vi "Calcy.vi"() -> ()   [LabVIEW 2025]
panel:
  in  "CLR":bool
  out "String":string
  in  "Keypad":T1
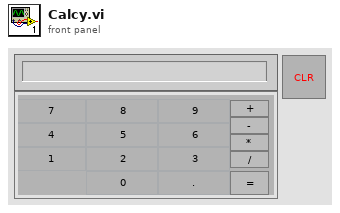
[diagram p1: front panel]
types:
  T1 = cluster{"0":bool, "1":bool, "2":bool, "3":bool, "4":bool, "5":bool, "6":bool, "7":bool, "8":bool, "9":bool, "decipoint":bool, "Add":bool, "Sub 3":bool, "Mul":bool, "Div":bool, "Equ":bool}
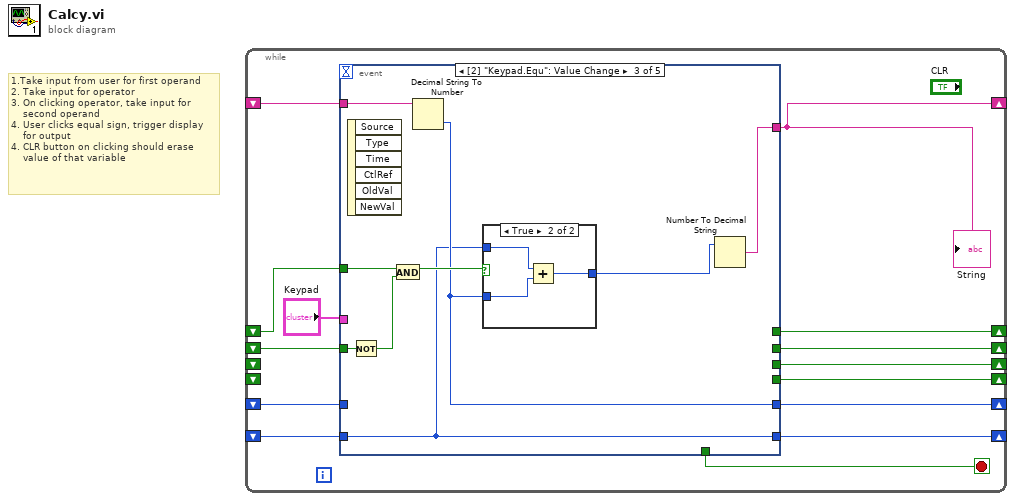
[diagram p0: block diagram]
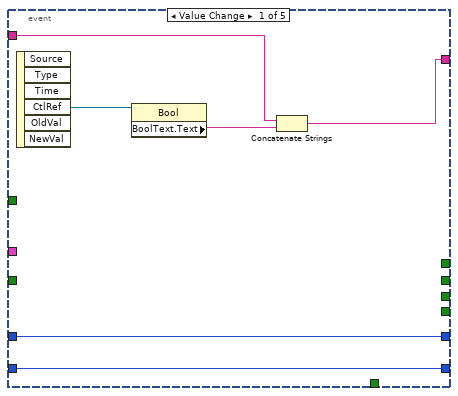
[diagram p2: hidden frame]
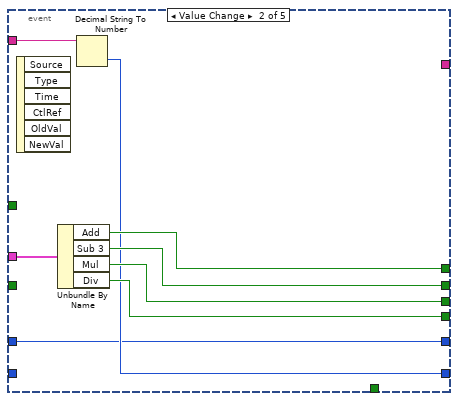
[diagram p3: hidden frame]
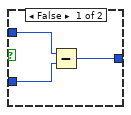
[diagram p4: hidden frame]
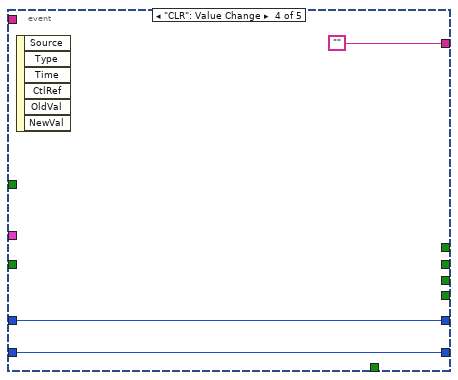
[diagram p5: hidden frame]
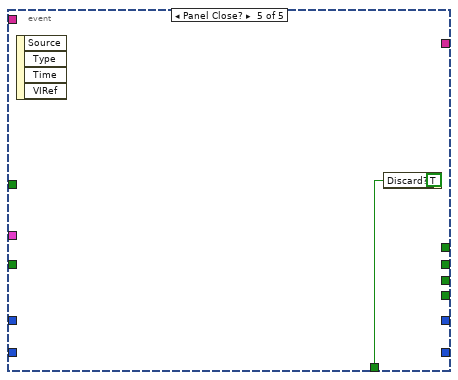
[diagram p6: hidden frame]
diagram:
  # "1.Take input from user for first operand\n2. Take input for operator\n3. On clicking operator, take input for\n    second operand\n4. User clicks equal sign, trigger display\n    for output\n4. CLR button on clicking should erase\n    value of that variable"
  n1 = while {
    shift-right: [w3] -> _
    shift-left: _ -> [w13]
    shift-right: [w12] -> _
    shift-left: _ -> [w11]
    shift-right: [w5] -> _
    shift-left: _ -> [w1]
    shift-right: [w6] -> _
    shift-left: _ -> [_]
    shift-right: [w4] -> _
    shift-left: _ -> [_]
    shift-right: [w7] -> _
    shift-left: _ -> [w2]
    shift-right: [w9] -> _
    shift-left: _ -> [w8]
    stop <- w14 stop-if-true
    n2 = event shown="[2] \"Keypad.Equ\": Value Change" {
      selector: _ -> [_ _ _ _ _]
      dyn-events: _ -> [_ _ _ _ _]
      timeout: _ -> [_ _ _ _ _]
      tunnel: [_ _ _ _ w47] -> w14
      tunnel: [w16 _ w37 "" _] -> w3
      tunnel: w13 -> [w18 w28 w36 _ _]
      tunnel: [w17 w22 w29 w45 _] -> w12
      tunnel: w11 -> [w17 _ w29 w45 _]
      tunnel: "Keypad" -> [_ w27 _ _ _]
      tunnel: [_ w23 _ _ _] -> w7
      tunnel: [_ w26 _ _ _] -> w5
      tunnel: [_ w25 _ _ _] -> w6
      tunnel: [_ w24 _ _ _] -> w4
      tunnel: [w15 w21 w30 w44 _] -> w9
      tunnel: w8 -> [w15 w21 _ w44 _]
      tunnel: w2 -> [_ _ w35 _ _]
      tunnel: w1 -> [_ _ w33 _ _]
      event "Keypad.1", "Keypad.2", "Keypad.3", "Keypad.4", "Keypad.5", "Keypad.6", "Keypad.7", "Keypad.8", "Keypad.9", "Keypad.0": Value Change {
        n3 = event-data() -> ("CtlRef"=w20:refnum<vi>)  [unwired: 1 in, 5 out]
        n4 = property class="Bool"(reference=w20) -> ("BoolText.Text"=w19:string)  [unwired: 1 in, 2 out]
        n5 = Concatenate Strings(w18, w19) -> (w16:string)
      }
      event "Keypad.Add", "Keypad.Sub 3", "Keypad.Mul", "Keypad.Div": Value Change {
        n6 = event-data() -> ()  [unwired: 1 in, 6 out]
        n7 = Unbundle By Name(w27) -> ("Add"=w23:bool, "Sub 3"=w26:bool, "Mul"=w25:bool, "Div"=w24:bool)
        n8 = Decimal String To Number(string=w28) -> (number=w22:i32)  [unwired: 2 in, 1 out]
      }
      event "Keypad.Equ": Value Change {
        n9 = event-data() -> ()  [unwired: 1 in, 6 out]
        n10 = Not(x=w33) -> (.not. x?=w32:bool)
        n11 = And(x=w35, y=w32) -> (x .and. y?=w34:bool)
        n12 = Decimal String To Number(string=w36) -> (number=w30:i32)  [unwired: 2 in, 1 out]
        n13 = case shown="True" w34 {
          tunnel: [w40 w43] -> w31
          tunnel: w30 -> [w38 w42]
          tunnel: w29 -> [w39 w41]
          frame False {
            n14 = Subtract(x=w39, y=w38) -> (x-y=w40:i32)
          }
          frame True {
            n15 = Add(x=w41, y=w42) -> (x+y=w43:i32)
          }
        }
        n16 = Number To Decimal String(number=w31) -> (decimal integer string=w37:string)  [unwired: 1 in]
      }
      event "CLR": Value Change {
        n17 = event-data() -> ()  [unwired: 1 in, 6 out]
      }
      event Panel Close? {
        w47 = TRUE ("Discard?")
        n18 = event-data() -> ()  [unwired: 1 in, 4 out]
        n19 = event-data("Discard?"=w47) -> ()  [unwired: 1 in, 1 out]
      }
    }
    "String" <- w3
  }
